vi "make xy voltage map.vi"() -> ()   [LabVIEW 2012]
uses:
  GFG/GFGnumericGet.vi
  GFG/GFGbooleanGet.vi
  GFG/GFG library.lvlib
panel:
  out "x voltage (after applying shift for Start.Delay)":T1(plugin-control)
  out "y voltage (after applying shift for Start.Delay)":T1(plugin-control)
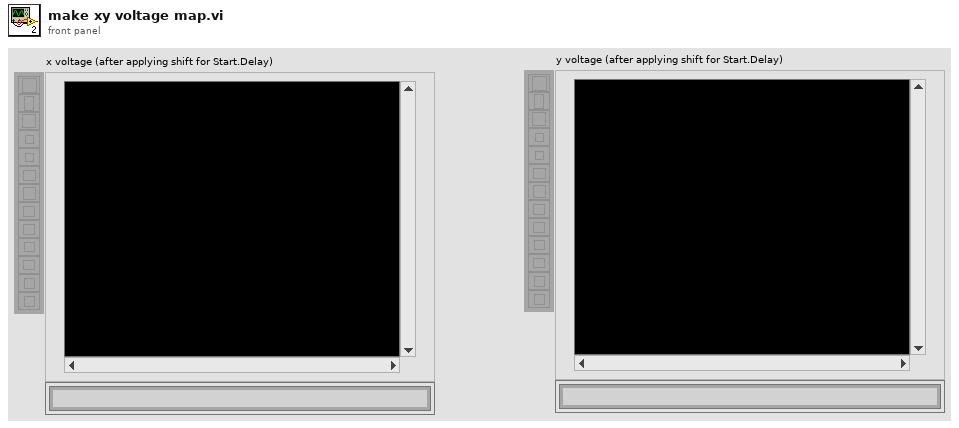
[diagram p1: front panel]
types:
  T1 = typedef "IMAQ Image.ctl" = refnum<image>
  T2 = typedef "Image Type" = u32
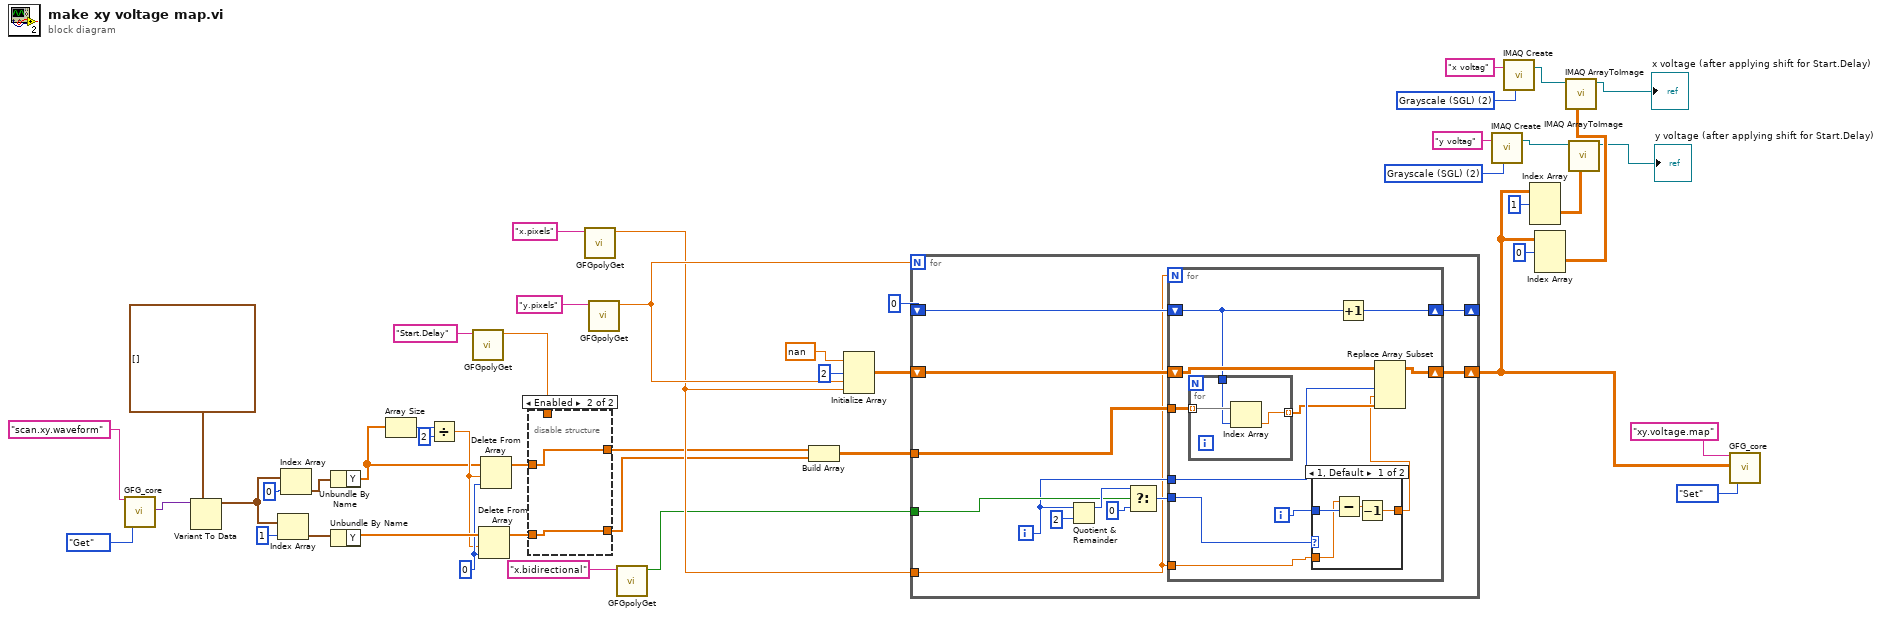
[diagram p0: block diagram]
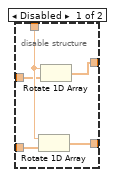
[diagram p2: hidden frame]
diagram:
  w10 = T2 2 items=["Grayscale (U8)", "Grayscale (I16)", "Grayscale (SGL)", "Complex (CSG)", "RGB (U32)", "HSL (U32)", "RGB (U64)", "Grayscale (U16)"] ("Image Type")
  w13 = T2 2 items=["Grayscale (U8)", "Grayscale (I16)", "Grayscale (SGL)", "Complex (CSG)", "RGB (U32)", "HSL (U32)", "RGB (U64)", "Grayscale (U16)"] ("Image Type")
  w27 = 0 ("index")
  n1 = call "GFG_core.vi"("Variable Name in"="scan.xy.waveform", "Action"=enum16{"Init", "Set", "Get"}."Get") -> ("Variant Out"=w16:variant)  [unwired: 11 in, 6 out]
  n2 = Variant To Data(type=waveform(dbl)[] [] ("frame scan geometry out"), Variant=w16) -> (data=w18:waveform(dbl)[])  [unwired: 1 in, 1 out]
  n3 = Index Array(array=w18, index=1) -> (element=w22:waveform(dbl))
  n4 = Index Array(array=w18, index=0) -> (element=w21:waveform(dbl))
  n5 = Unbundle By Name(w21) -> ("Y"=w25:dbl[])
  n6 = Unbundle By Name(w22) -> ("Y"=w28:dbl[])
  n7 = Array Size(array=w25) -> (size(s)=w23:i32)
  n8 = Divide(x=w23, y=2) -> (x/y=w26:dbl)
  n9 = call-poly "GFGpolyGet.vi"("Variable Name in"="Start.Delay") -> ("Numeric"=w32:dbl)  [unwired: 9 in, 1 out]
  n10 = Delete From Array(array=w28, length=w26, index=w27) -> (array with subset deleted=w31:dbl[])  [unwired: 1 out]
  n11 = Delete From Array(array=w25, length=w26, index=w27) -> (array with subset deleted=w29:dbl[])  [unwired: 1 out]
  n12 = disable-structure shown="Enabled" {
    disable-tunnel: [w52 w53] -> w41
    disable-tunnel: [w51 w54] -> w40
    disable-tunnel: w32 -> [w50 _]
    disable-tunnel: w31 -> [w49 w53]
    disable-tunnel: w29 -> [w48 w54]
    frame Disabled {
      n13 = Rotate 1D Array(1:w49, 2:w50) -> (0:w52:dbl[])
      n14 = Rotate 1D Array(1:w48, 2:w50) -> (0:w51:dbl[])
    }
    frame Enabled {
    }
  }
  n15 = call-poly "GFGpolyGet.vi"("Variable Name in"="x.pixels" ("Tag in")) -> ("Numeric"=w43:dbl)  [unwired: 9 in, 1 out]
  n16 = call-poly "GFGpolyGet.vi"("Variable Name in"="y.pixels" ("Tag in")) -> ("Numeric"=w44:dbl)  [unwired: 9 in, 1 out]
  n17 = call-poly "GFGpolyGet.vi"("Variable Name in"="x.bidirectional" ("Tag in")) -> ("Boolean"=w36:bool)  [unwired: 10 in]
  n18 = Build Array(w40, w41) -> (w42:dbl[][])
  n19 = Initialize Array(nan ("element"), 2 ("dimension size"), w44, w43) -> (w38:dbl[][][])
  n20 = for {
    N: w44 -> [_]
    tunnel: w43 -> [w56]
    tunnel: w36 -> [w62]
    shift-right: [w55] -> w3
    shift-left: w38 -> [w59]
    shift-right: [w60] -> _
    shift-left: 0 ("y") -> [w61]
    tunnel: w42 -> [w57]
    i -> [w58]
    n21 = Quotient & Remainder(x=w58, y=2) -> (x-y*floor(x/y)=w66:i32)  [unwired: 1 out]
    n22 = Select(t=w66, s=w62, f=0) -> (s? t:f=w63:i32)
    n23 = for {
      N: w56 -> [_]
      tunnel: w63 -> [w77]
      shift-right: [w76] -> w60
      shift-left: w61 -> [w69]
      shift-right: [w73] -> w55
      shift-left: w59 -> [w74]
      tunnel: w58 -> [w72]
      tunnel: w57 -> [w71]
      tunnel: w56 -> [w67]
      i -> [w75]
      n24 = for {
        tunnel: w71 -> [w80] mode=indexing
        tunnel: w69 -> [w79]
        tunnel: [w78] -> w70 mode=indexing
        n25 = Index Array(array=w80, index=w79) -> (element=w78:dbl)
      }
      n26 = case shown="1, Default" w77 {
        tunnel: w75 -> [w84 w85]
        tunnel: [w81 w85] -> w68
        tunnel: w67 -> [w83 _]
        frame 1, Default {
          n27 = Subtract(x=w83, y=w84) -> (x-y=w82:dbl)
          n28 = Decrement(x=w82) -> (x-1=w81:dbl)
        }
        frame 0 {
        }
      }
      n29 = Increment(x=w69) -> (x+1=w76:i32)
      n30 = Replace Array Subset(array=w74, new element=w70, index (dim 1)=w72, index (dim 2)=w68) -> (w73:dbl[][][])  [unwired: 1 in]
    }
  }
  n31 = call "IMAQ Create"("Image Name"="y voltag", "Image Type"=w10) -> ("New Image"=w8:T1)  [unwired: 3 in, 1 out]
  n32 = call "IMAQ Create"("Image Name"="x voltag", "Image Type"=w13) -> ("New Image"=w9:T1)  [unwired: 3 in, 1 out]
  n33 = Index Array(array=w3, index (dim 0)=1 ("index (page)")) -> (element=w2:dbl[][])  [unwired: 2 in]
  n34 = Index Array(array=w3, index (dim 0)=0 ("index (page)")) -> (element=w6:dbl[][])  [unwired: 2 in]
  n35 = call "IMAQ ArrayToImage"("Image Pixels (Float)"=w6, "Image"=w9) -> ("Image Out"=→"x voltage (after applying shift for Start.Delay)":T1)  [unwired: 8 in, 1 out]
  n36 = call "IMAQ ArrayToImage"("Image Pixels (Float)"=w2, "Image"=w8) -> ("Image Out"=→"y voltage (after applying shift for Start.Delay)":T1)  [unwired: 8 in, 1 out]
  n37 = call "GFG_core.vi"("Variable Name in"="xy.voltage.map", "Variant in"=w3, "Action"=enum16{"Init", "Set", "Get"}."Set") -> ()  [unwired: 10 in, 7 out]
